vi "enable_controls.vi"(8 "error in":errorcluster, 10 "Enable?":bool, 11 "Controls Label":string) -> (0 "error out":errorcluster)   [LabVIEW 2018]
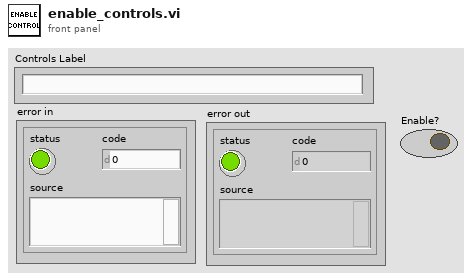
[diagram p1: front panel]
types:
  T1 = enum8{"Enabled", "Disabled", "Disabled and Grayed Out"}
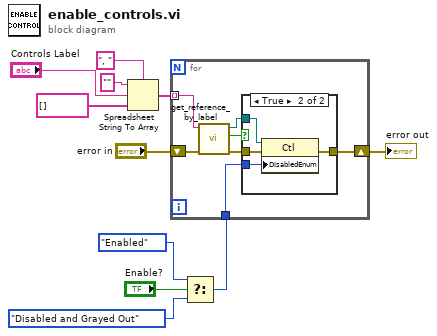
[diagram p0: block diagram]
diagram:
  n1 = Spreadsheet String To Array(delimiter (Tab)=", ", format string="", spreadsheet string="Controls Label", array type (2D Dbl)=string[] [] ("format string")) -> (array=w7:string[])
  n2 = Select(t=T1."Enabled" ("Disabled"), s="Enable?", f=T1."Disabled and Grayed Out" ("Disabled")) -> (s? t:f=w2:T1)
  n3 = for {
    tunnel: w7 -> [w18] mode=indexing
    shift-right: [w13] -> w1
    shift-left: "error in" -> [w17]
    tunnel: w2 -> [w12]
    n4 = call "get_reference_by_label.vi"("error in"=w17, "Label"=w18) -> ("error out"=w16:errorcluster, "Encontrado?"=w15:bool, "Ctl Refnum"=w14:refnum<vi>)  [unwired: 7 in]
    n5 = case shown="True" w15 {
      tunnel: w16 -> [w19 w22]
      tunnel: w14 -> [_ w23]
      tunnel: [w19 w21] -> w13
      tunnel: w12 -> [_ w20]
      frame False {
      }
      frame True {
        n6 = property class="Ctl"(reference=w23, error in=w22, "DisabledEnum"=w20) -> (error out=w21:errorcluster)  [unwired: 1 out]
      }
    }
  }
  "error out" <- w1
